vi "SFOAE-Create Concurrent Sweeps.vi"(0 "Sweep":T1, 5 "Concurrent":cluster{"Nsweeps":i32, "Overlap":dbl}, 7 "Level (dB SPL)":dbl, 9 "Cal File":path, 11 "error in (no error)":errorcluster, 12 "Fs (Hz)":dbl) -> (4 "sweep":dbl[](array[numeric]), 8 "offset":i32, 10 "nfft":i32, 15 "error out":errorcluster)   [LabVIEW 2020]
uses:
  Typedefs/SFOAE-Sweep Params.ctl
  <vilib>/Analysis/4window.llb/windowTd.ctl
  epl-vi-lib/PXI DAQ VIs/DAQ Engine VIs/PXI Globals.vi
  <vilib>/Analysis/NI_AALPro.lvlib
panel:
  out "size(s)":i32
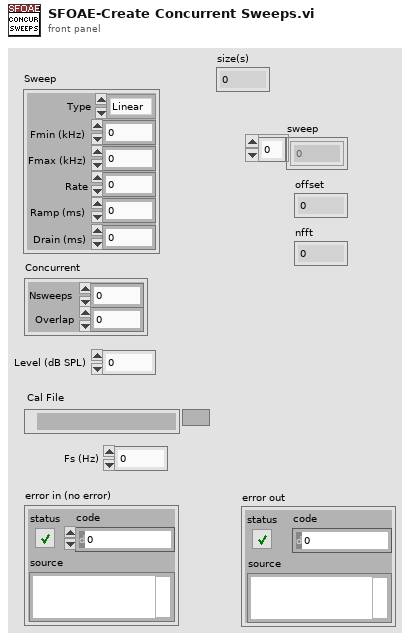
[diagram p1: front panel]
types:
  T1 = typedef "SFOAE-Sweep Params.ctl" = cluster{"Type":enum16{"Linear", "Log"}, "Fmin (kHz)":dbl, "Fmax (kHz)":dbl, "Rate":dbl, "Ramp (ms)":dbl, "Drain (ms)":dbl}
  T2 = typedef "NI_AALPro.lvlib/windowTd.ctl" = u32
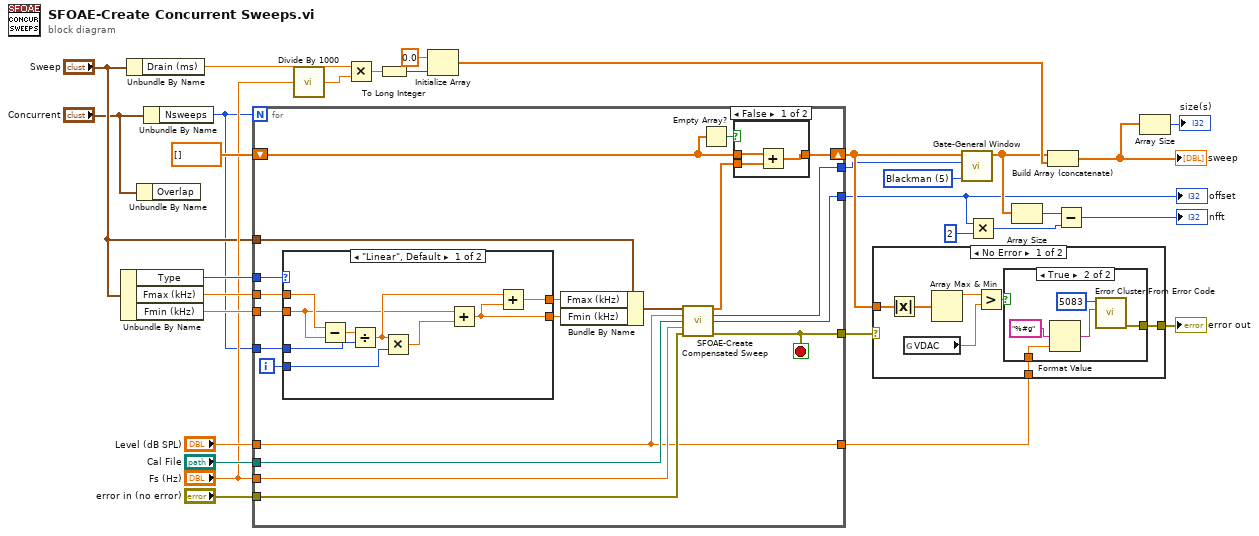
[diagram p0: block diagram]
diagram:
  w20 = T2 5 items=["Rectangle"=0, "Hanning"=1, "Hamming"=2, "Blackman-Harris"=3, "Exact Blackman"=4, "Blackman"=5, "Flat Top"=6, "4 Term B-Harris "=7, "7 Term B-Harris"=8, "Low Sidelobe"=9, "Blackman Nuttall"=11, "Triangle"=30, "Bartlett-Hanning"=31, "Bohman"=32, "Parzen"=33, "Welch"=34, "Kaiser"=60, "Dolph-Chebyshev"=61, "Gaussian"=62] ("window")
  n1 = Unbundle By Name("Sweep") -> ("Type"=w31:enum16{"Linear", "Log"}, "Fmax (kHz)"=w30:dbl, "Fmin (kHz)"=w29:dbl)
  n2 = Unbundle By Name("Sweep") -> ("Drain (ms)"=w16:dbl)
  n3 = Unbundle By Name("Concurrent") -> ()  [unwired: 1 out]
  n4 = Unbundle By Name("Concurrent") -> ("Nsweeps"=w7:i32)
  n5 = for {
    N: w7 -> [_]
    tunnel: w31 -> [w51]
    tunnel: w30 -> [w50]
    tunnel: w29 -> [w49]
    tunnel: w7 -> [w48]
    tunnel: "Sweep" -> [w46]
    tunnel: "Level (dB SPL)" -> [w37]
    tunnel: "Cal File" -> [w44]
    tunnel: "Fs (Hz)" -> [w43]
    tunnel: "error in (no error)" -> [w42]
    tunnel: [w41] -> w24
    shift-right: [w40] -> w21
    shift-left: dbl[] [] ("sweep") -> [w38]
    tunnel: [w37] -> w22
    tunnel: [w35] -> w6
    tunnel: [w32] -> w3
    i -> [w47]
    stop <- w41 stop-if-true
    n6 = case shown="\"Linear\", Default" w51 {
      tunnel: w50 -> [w64 _]
      tunnel: w49 -> [w57 _]
      tunnel: w48 -> [w62 _]
      tunnel: w47 -> [w58 _]
      tunnel: [w56 _] -> w36
      tunnel: [w60 _] -> w45
      frame "Linear", Default {
        n7 = Subtract(x=w64, y=w57) -> (x-y=w63:dbl)
        n8 = Divide(x=w63, y=w62) -> (x/y=w59:dbl)
        n9 = Multiply(x=w59, y=w58) -> (x*y=w61:dbl)
        n10 = Add(x=w57, y=w61) -> (x+y=w56:dbl)
        n11 = Add(x=w59, y=w56) -> (x+y=w60:dbl)
      }
      frame "Log" {
      }
    }
    n12 = Bundle By Name(cluster=w46, "Fmax (kHz)"=w45, "Fmin (kHz)"=w36) -> (w34:T1)
    n13 = call "SFOAE-Create Compensated Sweep.vi"("Sweep"=w34, "Level (dB SPL)"=w37, "Cal File"=w44, "Fs (Hz)"=w43, "error in (no error)"=w42) -> ("sweep"=w33:dbl[], "RampPts"=w32:i32, "offset"=w35:i32, "error out"=w41:errorcluster)  [unwired: 7 in]
    n14 = Empty Array?(array=w38) -> (empty?=w39:bool)
    n15 = case shown="False" w39 {
      tunnel: w33 -> [w52 w55]
      tunnel: [w53 w55] -> w40
      tunnel: w38 -> [w54 _]
      frame False {
        n16 = Add(x=w54, y=w52) -> (x+y=w53:dbl[])
      }
      frame True {
      }
    }
  }
  "offset" <- w6
  n17 = call "Divide By 1000.vi"("X"="Fs (Hz)") -> ("X/1000"=w17:dbl)
  n18 = Multiply(x=w16, y=w17) -> (x*y=w15:dbl)
  n19 = To Long Integer(number=w15) -> (32bit integer=w14:i32)
  n20 = Initialize Array(0.0 ("element"), w14) -> (w12:dbl[])
  n21 = case shown="No Error" w24 {
    selector: w24 -> [_ w77]
    tunnel: [w66 w77] -> w23
    tunnel: w21 -> [w71 _]
    tunnel: w22 -> [w65 _]
    frame No Error {
      n22 = Absolute Value(x=w71) -> (abs(x)=w70:dbl[])
      n23 = global read "PXI Globals.vi" "VDAC"() -> (w68:dbl)
      n24 = Array Max & Min(array=w70) -> (max value=w69:dbl)  [unwired: 3 out]
      n25 = Greater?(x=w69, y=w68) -> (0:w67:bool)
      n26 = case shown="True" w67 {
        tunnel: [_ w76] -> w66
        tunnel: w65 -> [_ w73]
        frame False {
        }
        frame True {
          n27 = Format Value(format string="%#g", value (0)=w73) -> (output string=w74:string)  [unwired: 1 in]
          n28 = call <vilib>:"Error Cluster From Error Code.vi"("error message (\"\")"=w74, "error code (0)"=5083) -> ("error out"=w76:errorcluster)  [unwired: 7 in]
        }
      }
    }
    frame Error {
    }
  }
  "error out" <- w23
  n29 = call "Gate-General Window.vi"("window"=w20, "Nramp"=w3, "X"=w21) -> ("X windowed"=w11:dbl[])  [unwired: 8 in]
  n30 = Multiply(x=w6, y=2) -> (x*y=w9:i32)
  n31 = Array Size(array=w11) -> (size(s)=w10:i32)
  n32 = Build Array (concatenate)(w11, w12) -> (w2:dbl[])
  "sweep" <- w2
  n33 = Subtract(x=w10, y=w9) -> (x-y=→"nfft":i32)
  n34 = Array Size(array=w2) -> (size(s)=→"size(s)":i32)
